vi "se1e1.vi"(0 "A":dbl, 1 "B":dbl) -> (2 "Numeric 2":dbl, 3 "Numeric":dbl, 4 "x = y?":bool)   [LabVIEW 2013]
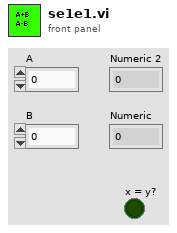
[diagram p1: front panel]
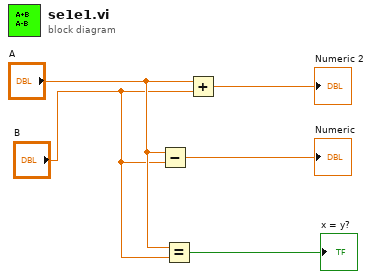
[diagram p0: block diagram]
diagram:
  n1 = Subtract(x="A", y="B") -> (x-y=→"Numeric":dbl)
  n2 = Equal?(x="A", y="B") -> (x = y?=→"x = y?":bool)
  n3 = Add(x="A", y="B") -> (x+y=→"Numeric 2":dbl)
